vi "Get_Y.vi"(8 "error in (no error)":errorcluster caption="错误输入（无错误）", 11 "Point输入":refnum<class "Point.lvclass">) -> (0 "error out":errorcluster caption="错误输出", 2 "Y":dbl, 3 "Point输出":refnum<class "Point.lvclass">)   [LabVIEW 2011, in "Point.lvclass"]
uses:
  Point.lvclass
  Point.lvclass/Point.ctl
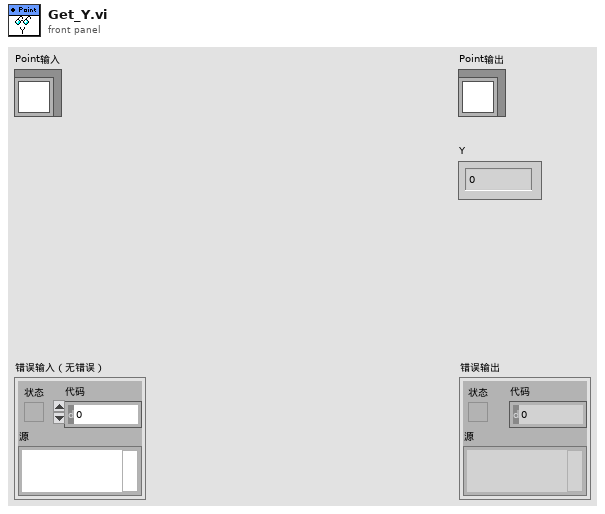
[diagram p1: front panel]
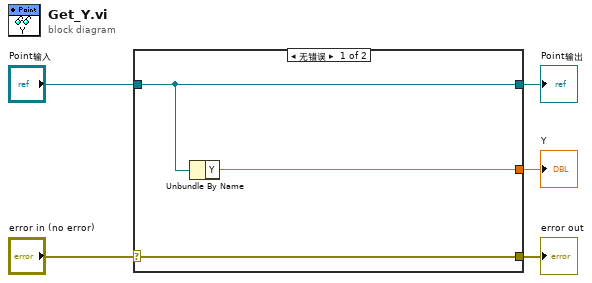
[diagram p0: block diagram]
diagram:
  n1 = case shown="无错误" "error in (no error)" {
    selector: "error in (no error)" -> [w8 w9]
    tunnel: [w8 w9] -> w4
    tunnel: [w7 w10] -> w2
    tunnel: "Point输入" -> [w7 w10]
    tunnel: [w6 _] -> w1
    frame No Error {
      n2 = Unbundle By Name(w7) -> ("Y"=w6:dbl)
    }
    frame Error {
    }
  }
  "error out" <- w4
  "Point输出" <- w2
  "Y" <- w1
